vi "getDigitalValue.vi"(8 "error in (no error)":errorcluster, 11 "ScriptEvent in":refnum<class "ScriptEvent.lvclass">) -> (0 "error out":errorcluster, 2 "digitalValue":dbl, 3 "ScriptEvent out":refnum<class "ScriptEvent.lvclass">)   [LabVIEW 2011, in "Tools.lvlib" / "Scripting.lvlib" / "ScriptEvent.lvclass"]
uses:
  ScriptEvent.lvclass
  DatabaseHelpers/Database Objects/Channel/DigitalChannel/DigitalChannel.lvclass
  ScriptEvent.lvclass/ScriptEvent.ctl
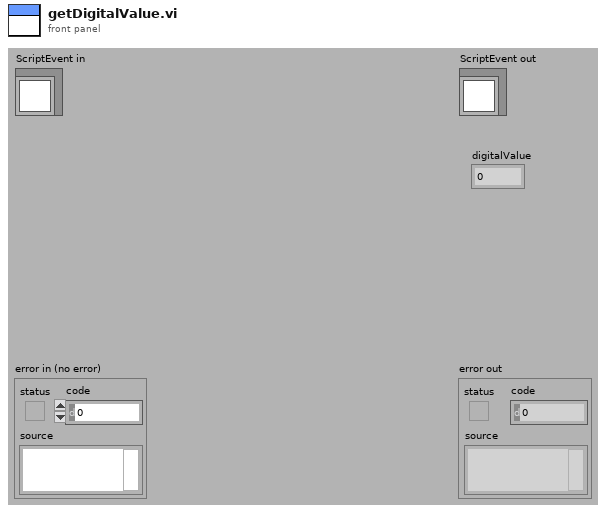
[diagram p1: front panel]
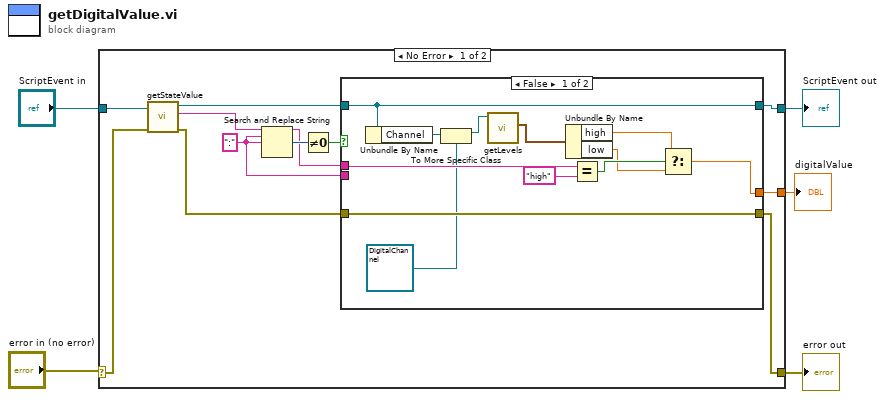
[diagram p0: block diagram]
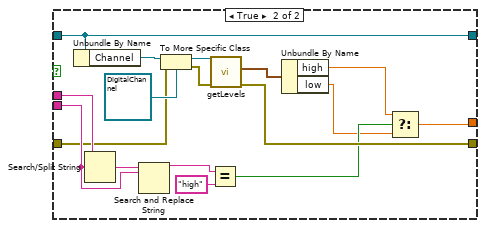
[diagram p2: hidden frame]
diagram:
  n1 = case shown="No Error" "error in (no error)" {
    selector: "error in (no error)" -> [w11 w48]
    tunnel: [w6 w48] -> w4
    tunnel: [w8 w47] -> w2
    tunnel: "ScriptEvent in" -> [w12 w47]
    tunnel: [w7 _] -> w1
    frame No Error {
      w13 = ":"
      n2 = call-dynamic "getStateValue.vi"("error in (no error)"=w11, "ScriptEvent in"=w12) -> ("error out"=w9:errorcluster, "stateValue"=w17:string, "ScriptEvent out"=w10:refnum<class "ScriptEvent.lvclass">)  [unwired: 7 in]
      n3 = Search and Replace String(input string=w17, search string=w13, replace string=w13) -> (result string=w14:string, number of replacements=w16:i32)  [unwired: 5 in, 2 out]
      n4 = Not Equal To 0?(x=w16) -> (x != 0?=w15:bool)
      n5 = case shown="False" w15 {
        tunnel: w14 -> [w28 w46]
        tunnel: w13 -> [_ w44]
        tunnel: [w18 w30] -> w7
        tunnel: w10 -> [w25 w37]
        tunnel: w9 -> [w29 w39]
        tunnel: [w29 w38] -> w6
        tunnel: [w25 w37] -> w8
        frame False {
          n6 = Unbundle By Name(w25) -> ("Channel"=w24:refnum<class "Channel.lvclass">)
          n7 = To More Specific Class(target class=refnum<class "DigitalChannel.lvclass"> refnum ("DigitalChannel.lvclass in"), reference=w24) -> (specific class reference=w23:refnum<class "DigitalChannel.lvclass">)  [unwired: 1 in, 1 out]
          n8 = call "getLevels.vi"("DigitalChannel.lvclass in"=w23) -> ("levels"=w21:cluster{"high":dbl, "low":dbl})  [unwired: 8 in, 2 out]
          n9 = Unbundle By Name(w21) -> ("high"=w20:dbl, "low"=w19:dbl)
          n10 = Equal?(x=w28, y="high") -> (x = y?=w26:bool)
          n11 = Select(t=w20, s=w26, f=w19) -> (s? t:f=w18:dbl)
        }
        frame True {
          n12 = Unbundle By Name(w37) -> ("Channel"=w43:refnum<class "Channel.lvclass">)
          n13 = Search/Split String(string=w46, search string/char (-)=w44) -> (match + rest of string=w45:string)  [unwired: 1 in, 2 out]
          n14 = Search and Replace String(input string=w45, search string=w44) -> (result string=w34:string)  [unwired: 6 in, 3 out]
          n15 = To More Specific Class(target class=refnum<class "DigitalChannel.lvclass"> refnum ("Tools.lvlib:DatabaseHelpers.lvlib:DigitalChannel.lvclass"), reference=w43, error in=w39) -> (specific class reference=w41:refnum<class "DigitalChannel.lvclass">, error out=w40:errorcluster)
          n16 = Equal?(x=w34, y="high") -> (x = y?=w32:bool)
          n17 = call "getLevels.vi"("error in (no error)"=w40, "DigitalChannel.lvclass in"=w41) -> ("error out"=w38:errorcluster, "levels"=w36:cluster{"high":dbl, "low":dbl})  [unwired: 7 in, 1 out]
          n18 = Unbundle By Name(w36) -> ("high"=w33:dbl, "low"=w31:dbl)
          n19 = Select(t=w33, s=w32, f=w31) -> (s? t:f=w30:dbl)
        }
      }
    }
    frame Error {
    }
  }
  "error out" <- w4
  "ScriptEvent out" <- w2
  "digitalValue" <- w1
